vi "CLD 14 Timer Application Exercise.vi"() -> ()   [LabVIEW 2009]
panel:
  out "Zielzeit (s)":dbl
  out "Verstrichene Zeit (s)":dbl
  in  "Stopp":bool
  in  "Anhalten":bool
  in  "Abbrechen":bool
  in  "Start":bool
  in  "Fehler (Eingang)":errorcluster
  out "Fehler (Ausgang)":errorcluster
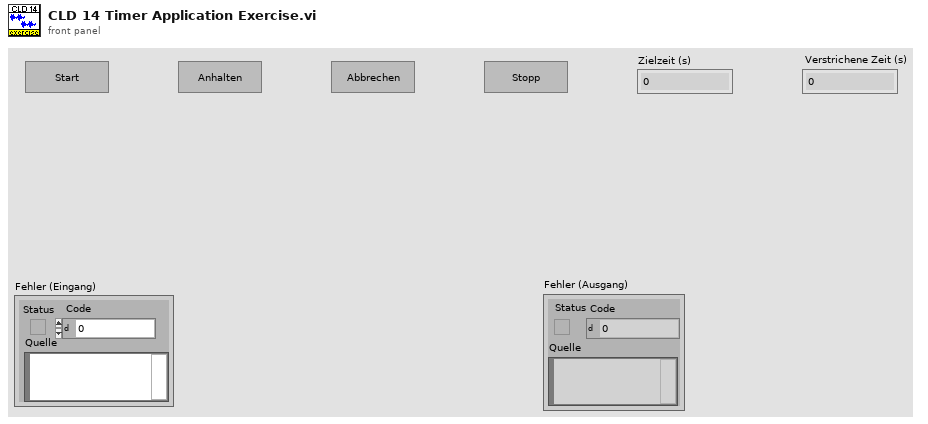
[diagram p1: front panel]
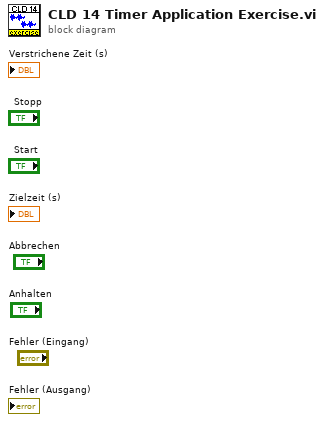
[diagram p0: block diagram]
diagram:
